vi "test Remove Only Alias In List.vi"(8 "error in (no error)":errorcluster, 11 "TestCase in":refnum<class "Routing and Faulting Aliases Unit Tests.lvclass">) -> (0 "error out":errorcluster, 3 "TestCase out":refnum<class "Routing and Faulting Aliases Unit Tests.lvclass">)   [LabVIEW 2017, in "Routing and Faulting Aliases Unit Tests.lvclass"]
uses:
  Routing and Faulting Aliases Unit Tests.lvclass
  System Explorer/Alias.ctl
  System Explorer/Endpoint.ctl
  Routing and Faulting Aliases Unit Tests.lvclass/Routing and Faulting Aliases Unit Tests.ctl
  <vilib>/addons/_JKI Toolkits/VI Tester/TestCase.llb/TestCase.lvclass
  System Explorer/Routing and Faulting System Explorer.lvlib
  Scripting/Routing and Faulting Scripting.lvlib
  C:/Program Files (x86)/National Instruments/LabVIEW 2017/vi.lib/addons/_JKI Toolkits/VI Tester/TestCase.llb/TestCase.lvclass
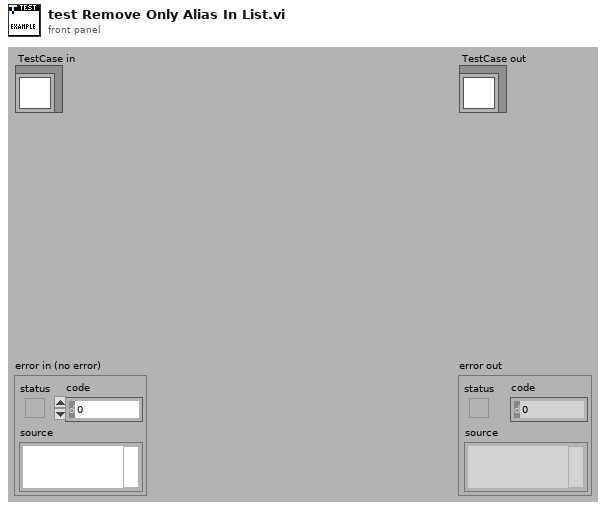
[diagram p1: front panel]
types:
  T1 = typedef "Routing and Faulting System Explorer.lvlib/Alias.ctl" = cluster{"Endpoint":T2, "Alias":string, "Remove":bool}
  T2 = typedef "Routing and Faulting System Explorer.lvlib/Endpoint.ctl" = string
  T3 = typedef "Custom Device API.lvlib/Custom Device Item Ref.ctl" = u64
  T4 = typedef "Routing and Faulting Shared.lvlib/Alias Mapping.ctl" = cluster{"Endpoint":string, "Alias":string}
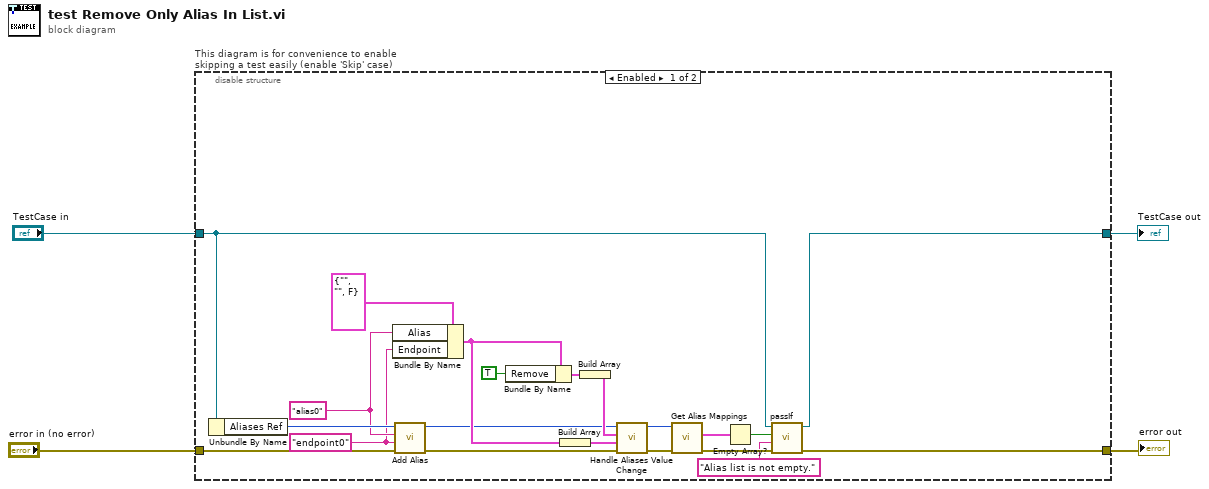
[diagram p0: block diagram]
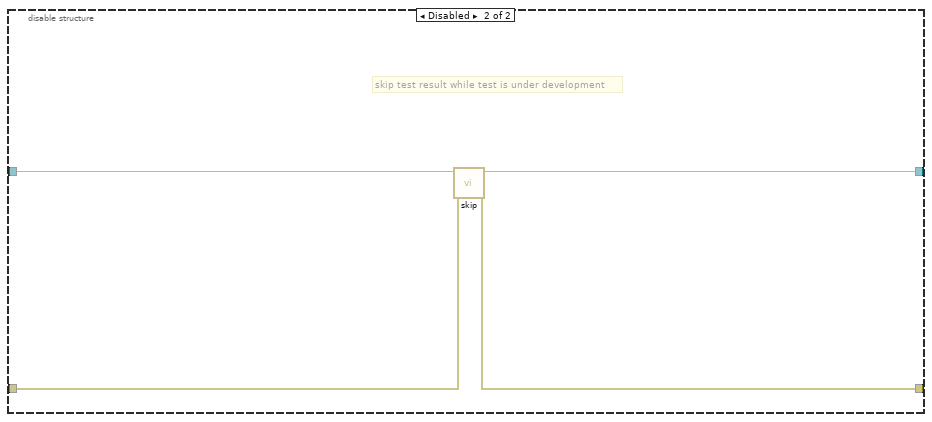
[diagram p2: hidden frame]
diagram:
  n1 = disable-structure "This diagram is for convenience to enable skipping a test easily (enable 'Skip' case)" shown="Enabled" {
    disable-tunnel: "TestCase in" -> [w21 w29]
    disable-tunnel: [w20 w27] -> w1
    disable-tunnel: [w22 w28] -> w3
    disable-tunnel: "error in (no error)" -> [w19 w26]
    frame Enabled {
      w14 = "endpoint0" ("Endpoint")
      w15 = "alias0" ("Alias")
      n2 = Unbundle By Name(w21) -> ("Aliases Ref"=w18:T3)
      n3 = Bundle By Name(cluster=T1 {"Endpoint"="", "Alias"="", "Remove"=FALSE} ("Alias"), "Alias"=w15, "Endpoint"=w14) -> (w10:T1)
      n4 = call "Add Alias.vi"("error in (no error)"=w19, "Endpoint"=w14, "Alias"=w15, "Endpoint Aliases Ref in"=w18) -> ("error out"=w17:errorcluster, "Endpoint Aliases Ref out"=w5:T3)  [unwired: 6 in]
      n5 = Bundle By Name(cluster=w10, "Remove"=TRUE) -> (w12:T1)
      n6 = Build Array(w10) -> (w9:T1[])
      n7 = Build Array(w12) -> (w11:T1[])
      n8 = call "Handle Aliases Value Change.vi"("error in (no error)"=w17, "OldVal"=w9, "NewVal"=w11, "Aliases Ref in"=w5) -> ("error out"=w25:errorcluster, "Aliases Ref out"=w24:T3)  [unwired: 6 in]
      n9 = call "Get Alias Mappings.vi"("error in (no error)"=w25, "Endpoint Aliases Ref in"=w24) -> ("error out"=w23:errorcluster, "Alias Mappings"=w8:T4[])  [unwired: 7 in, 1 out]
      n10 = Empty Array?(array=w8) -> (empty?=w7:bool)
      n11 = call-dynamic "passIf.vi"("error in (no error)"=w23, "message (\"\")"="Alias list is not empty." ("message (\"\")"), "pass"=w7, "TestCase in"=w21) -> ("error out"=w22:errorcluster, "TestCase out"=w20:refnum<class "Routing and Faulting Aliases Unit Tests.lvclass">)  [unwired: 6 in]
    }
    frame Disabled {
      # "skip test result while test is under development"
      n12 = call <vilib>:"skip.vi"("error in (no error)"=w26, "TestCase in"=w29) -> ("error out"=w28:errorcluster, "TestCase out"=w27:refnum<class "Routing and Faulting Aliases Unit Tests.lvclass">)  [unwired: 8 in]
    }
  }
  "error out" <- w3
  "TestCase out" <- w1
